vi "Write Channel Data with Headers.vi"() -> ()   [LabVIEW 2018]
uses:
  <vilib>/Analysis/NI_AALBase.lvlib
panel:
  in  "Channel 1 Name":string="Test Data 1"
  in  "Channel 0 Name":string="Test Data 2"
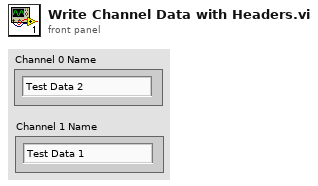
[diagram p1: front panel]
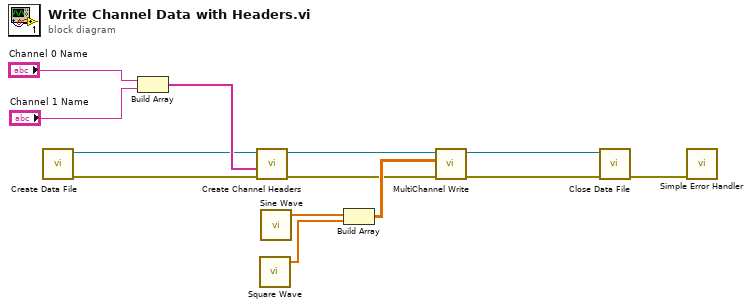
[diagram p0: block diagram]
diagram:
  n1 = call "Create Data File.vi"() -> ("Error Out"=w7:errorcluster, "File Refnum"=w6:refnum<file>)  [unwired: 10 in]
  n2 = Build Array("Channel 0 Name", "Channel 1 Name") -> (w8:string[])
  n3 = call "Create Channel Headers.vi"("Error In"=w7, "Channel Names"=w8, "File Refnum In"=w6) -> ("Error Out"=w2:errorcluster, "File Refnum Out"=w5:refnum<file>)  [unwired: 7 in]
  n4 = call <vilib>:"Square Wave.vi"() -> ("square wave"=w11:dbl[])  [unwired: 6 in, 2 out]
  n5 = call <vilib>:"Sine Wave.vi"() -> ("sine wave"=w12:dbl[])  [unwired: 5 in, 2 out]
  n6 = Build Array(w12, w11) -> (w3:dbl[][])
  n7 = call "MultiChannel Write.vi"("Error In"=w2, "Data to Log"=w3, "File Refnum In"=w5) -> ("Error Out"=w1:errorcluster, "File Refnum Out"=w4:refnum<file>)  [unwired: 7 in]
  n8 = call "Close Data File.vi"("error in"=w1, "File Refnum In"=w4) -> ("error out"=w13:errorcluster)  [unwired: 9 in]
  n9 = call <vilib>:"Simple Error Handler.vi"("error in (no error)"=w13) -> ()  [unwired: 4 in, 5 out]
